vi "RH_FGEN_Configure.vi"(6 "Marker Position":i32, 7 "FGEN Parameters":T2 {"Trigger Mode" items=["Single", "Continuous", "Stepped", "Burst"]}, 8 "error in":errorcluster, 9 "Output Terminal (do not export)":T1, 10 "Channel Name":string, 11 "FGEN Session In":refnum<k15>) -> (0 "error out":errorcluster, 3 "FGEN Session Out":refnum<k15>)   [LabVIEW 2023, in "ResourceHandling.lvlib"]
doc: "Configure the resource in Arbitrary Waveform mode, setting Marker 0 and exporting it to PXI_Trig lines"
uses:
  ResourceHandling.lvlib
  TypeDefs/RH_FGEN_Parameters.ctl
  <instrlib>/niFgen/niFgen.llb/niFgen Trigger Mode.ctl
  <instrlib>/niFgen/niFgen.llb/niFgen_ctl Exported Signal Desination Values (ComboBox).ctl
  <instrlib>/niFgen/niFgen.llb/niFgen Output Mode.ctl
  <instrlib>/niFgen/niFgen.llb/niFgen_ctl Exported Signal Name Values (Ring).ctl
  <instrlib>/niFgen/niFgen.llb/niFgen_ctl Exported Signal Identifiers (Ring).ctl
  <instrlib>/niFgen/niFgen.llb/niFgen Disable Start Trigger.vi
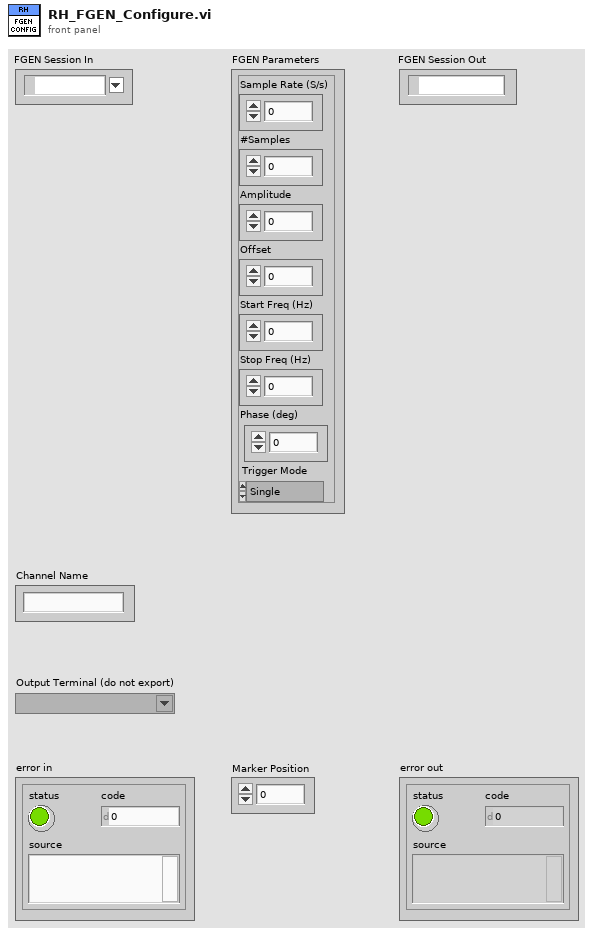
[diagram p1: front panel]
types:
  T1 = typedef "niFgen_ctl Exported Signal Desination Values (ComboBox).ctl" = string
  T2 = typedef "ResourceHandling.lvlib/RH_FGEN_Parameters.ctl" = cluster{"Sample Rate (S/s)":dbl, "#Samples":i32, "Amplitude":dbl, "Offset":dbl, "Start Freq (Hz)":dbl, "Stop Freq (Hz)":dbl, "Phase (deg)":dbl, "Trigger Mode":T3}
  T3 = typedef "niFgen Trigger Mode.ctl" = i32
  T4 = typedef "niFgen_ctl Exported Signal Identifiers (Ring).ctl" = string
  T5 = typedef "niFgen_ctl Exported Signal Name Values (Ring).ctl" = u16
  T6 = typedef "niFgen Output Mode.ctl" = u32
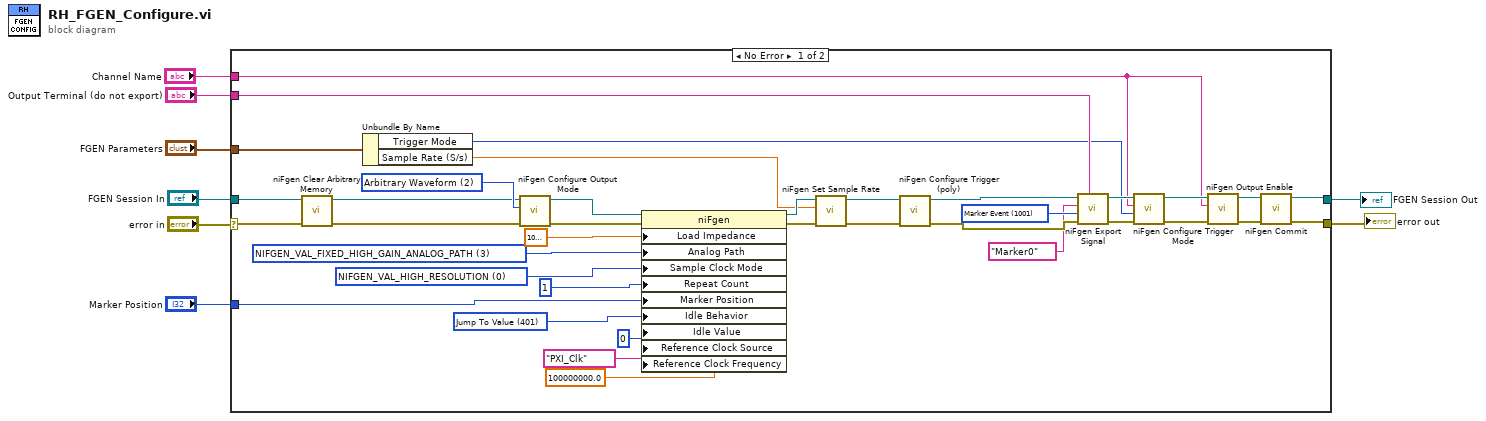
[diagram p0: block diagram]
diagram:
  n1 = case shown="No Error" "error in" {
    selector: "error in" -> [w26 w47]
    tunnel: "FGEN Parameters" -> [w30 _]
    tunnel: "FGEN Session In" -> [w25 w46]
    tunnel: [w12 w47] -> w2
    tunnel: [w11 w46] -> w3
    tunnel: "Output Terminal (do not export)" -> [w29 _]
    tunnel: "Channel Name" -> [w10 _]
    tunnel: "Marker Position" -> [w9 _]
    frame No Error {
      w21 = T5 1001 items=["Sample Clock"=101, "Sample Clock Timebase"=1006, "Reference Clock"=102, "Onboard Reference Clock"=1019, "Start Trigger"=1004, "Script Trigger"=103, "Marker Event"=1001, "Data Marker Event"=108, "Ready For Start Event"=105, "Started Event"=106, "Done Event"=107, "Synchronization Pulse"=1007, "Sync Out"=1002] ("Signal")
      w33 = 401 items=["Hold Last Value"=400, "Jump To Value"=401] ("Output:Advanced:Idle Behavior")
      w36 = T6 2 items=["Standard Function", "Frequency List", "Arbitrary Waveform", "Arbitrary Sequence", "Script"] ("Output Mode (default: 0=Standard Function)")
      w37 = 3 items=["NIFGEN_VAL_MAIN_ANALOG_PATH", "NIFGEN_VAL_DIRECT_ANALOG_PATH", "NIFGEN_VAL_FIXED_LOW_GAIN_ANALOG_PATH", "NIFGEN_VAL_FIXED_HIGH_GAIN_ANALOG_PATH"] ("Output:Analog Path")
      w40 = 0 items=["NIFGEN_VAL_DIVIDE_DOWN"=1, "NIFGEN_VAL_HIGH_RESOLUTION"=0, "NIFGEN_VAL_AUTOMATIC"=2] ("Clocks:Sample Clock:Mode")
      n2 = call <instrlib>:"niFgen Clear Arbitrary Memory.vi"("error in (no error)"=w26, "Instrument Handle"=w25) -> ("error out"=w27:errorcluster, "Instrument Handle Out"=w28:refnum<k15>)  [unwired: 8 in]
      n3 = Unbundle By Name(w30) -> ("Trigger Mode"=w17:T3, "Sample Rate (S/s)"=w41:dbl)
      n4 = call <instrlib>:"niFgen Configure Output Mode.vi"("error in (no error)"=w27, "Output Mode (default: 0=Standard Function)"=w36, "Instrument Handle"=w28) -> ("error out"=w44:errorcluster, "Instrument Handle Out"=w45:refnum<k15>)  [unwired: 6 in]
      n5 = property class="niFgen"(reference=w45, error in=w44, "Load Impedance"=1000000.0 ("Output:Load Impedance"), "Analog Path"=w37, "Sample Clock Mode"=w40, "Repeat Count"=1 ("Arbitrary Waveform:Arbitrary Waveform Mode:Repeat Count"), "Marker Position"=w9, "Idle Behavior"=w33, "Idle Value"=0 ("Output:Advanced:Idle Value"), "Reference Clock Source"="PXI_Clk" ("Clocks:Reference Clock:Source"), "Reference Clock Frequency"=100000000.0 ("Clocks:Reference Clock:Frequency")) -> (reference out=w43:refnum<k15>, error out=w42:errorcluster)
      n6 = call <instrlib>:"niFgen Set Sample Rate.vi"("error in (no error)"=w42, "Sample Rate (Samp/s)"=w41, "Instrument Handle"=w43) -> ("error out"=w35:errorcluster, "Instrument Handle Out"=w34:refnum<k15>)  [unwired: 7 in]
      n7 = call-poly <instrlib>:"niFgen Configure Trigger (poly).vi"("error in (no error)"=w35, "Instrument Handle"=w34) -> ("error out"=w22:errorcluster, "Instrument Handle Out"=w23:refnum<k15>)  [unwired: 8 in]
      n8 = call <instrlib>:"niFgen Export Signal.vi"("Output Terminal (do not export)"=w29, "error in (no error)"=w22, "Signal"=w21, "Signal Identifier (None)"=T4 "Marker0", "Instrument Handle"=w23) -> ("error out"=w19:errorcluster, "Instrument Handle Out"=w18:refnum<k15>)  [unwired: 5 in]
      n9 = call <instrlib>:"niFgen Configure Trigger Mode.vi"("error in (no error)"=w19, "Trigger Mode (default: 1=continuous)"=w17, "Channel Name"=w10, "Instrument Handle"=w18) -> ("error out"=w16:errorcluster, "Instrument Handle Out"=w15:refnum<k15>)  [unwired: 6 in]
      n10 = call <instrlib>:"niFgen Output Enable.vi"("error in (no error)"=w16, "Channel Name"=w10, "Instrument Handle"=w15) -> ("error out"=w14:errorcluster, "Instrument Handle Out"=w13:refnum<k15>)  [unwired: 7 in]
      n11 = call <instrlib>:"niFgen Commit.vi"("error in (no error)"=w14, "Instrument Handle"=w13) -> ("error out"=w12:errorcluster, "Instrument Handle Out"=w11:refnum<k15>)  [unwired: 8 in]
    }
    frame Error {
    }
  }
  "FGEN Session Out" <- w3
  "error out" <- w2
